vi "DSDLL Cleanup Digitizing Process.vi"(8 "error in":errorcluster, 11 "dsdll in":T1) -> (0 "error out":errorcluster, 3 "dsdll out":T1)   [LabVIEW 2018, in "DSDLL Virtual Digitizer.lvlib"]
doc: "Cleans up everything related to the digitizing process. Must be called after each use of Initiate Digitizing Process to deallocate all related objects and to stop Digitizing Process. It must be called even if digitizing failed or was aborted!\nThe VI ignores input error so it will always execute."
uses:
  DSDLL Virtual Digitizer.lvlib
  DSDLL Session.ctl
  dsdll source distribution/dsdll_instance.ctl
  dsdll source distribution/dsdll_device_record.ctl
  DSDLL Process Config.ctl
  DSDLL Data Packet.ctl
  dsdll source distribution/dsdll.lvlib
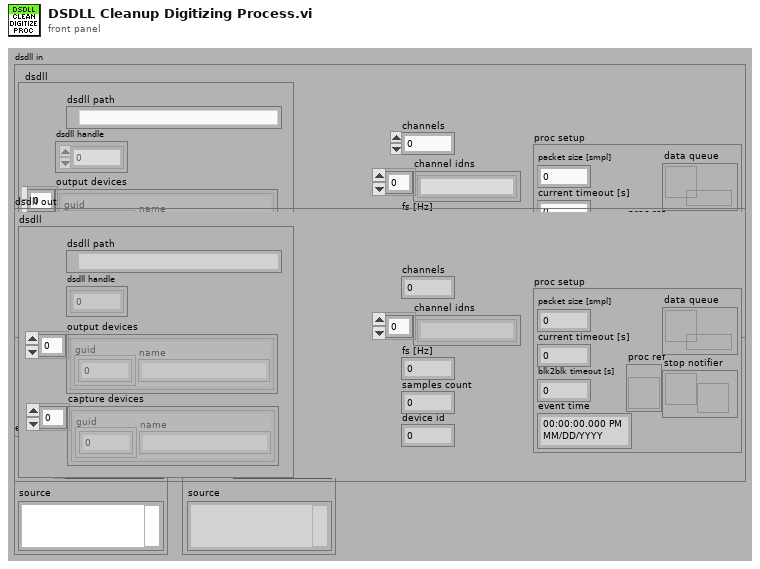
[diagram p1: front panel]
types:
  T1 = typedef "DSDLL Virtual Digitizer.lvlib/DSDLL Session.ctl" = cluster{"dsdll":T2, "channels":i32, "device id":i32, "channel idns":string[], "proc setup":T4, "samples count":i32, "fs [Hz]":dbl}
  T2 = typedef "dsdll.lvlib/dsdll_instance.ctl" = cluster{"dsdll path":path, "dsdll handle":u8[], "output devices":T3[], "capture devices":T3[]}
  T3 = typedef "dsdll.lvlib/dsdll_device_record.ctl" = cluster{"guid":u8[], "name":string}
  T4 = typedef "DSDLL Virtual Digitizer.lvlib/DSDLL Process Config.ctl" = cluster{"packet size [smpl]":i32, "current timeout [s]":dbl, "blk2blk timeout [s]":dbl, "event time":timestamp, "data queue":refnum<queue>, "stop notifier":refnum<notifier>, "proc ref":refnum<vi>}
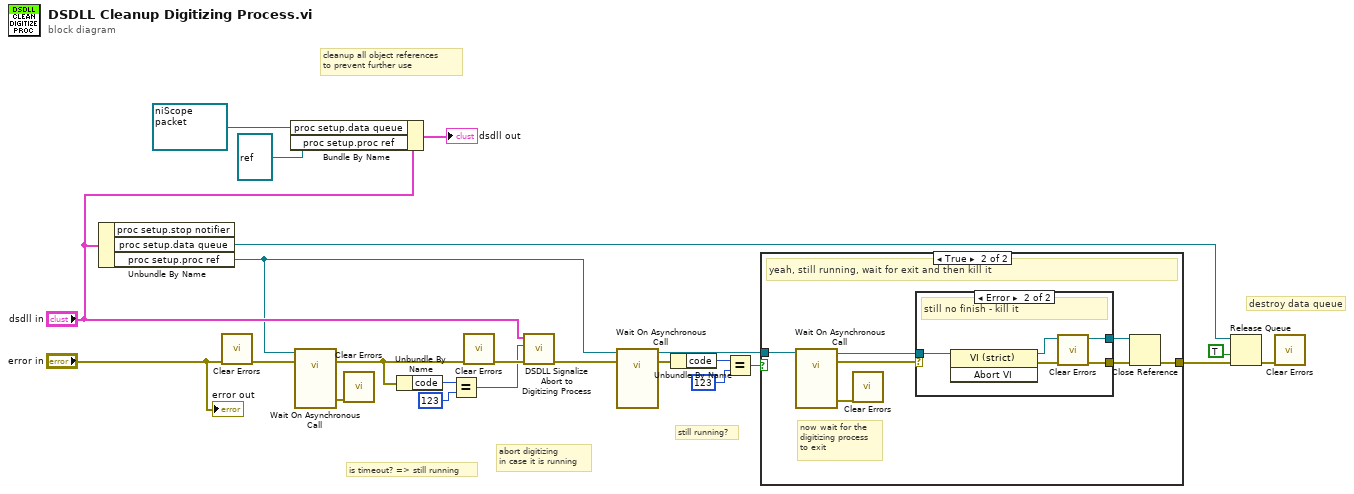
[diagram p0: block diagram]
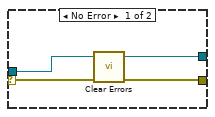
[diagram p3: hidden frame]
diagram:
  # "still running?"
  # "abort digitizing\nin case it is running"
  # "cleanup all object references\nto prevent further use"
  # "destroy data queue"
  # "is timeout? => still running"
  n1 = Unbundle By Name("dsdll in") -> ("proc setup.data queue"=w20:refnum<queue>, "proc setup.proc ref"=w7:refnum<vi>)  [unwired: 1 out]
  n2 = call <vilib>:"Clear Errors.vi"("error in (no error)"="error in") -> ("error out"=w14:errorcluster)  [unwired: 5 in, 1 out]
  n3 = Bundle By Name(cluster="dsdll in", "proc setup.data queue"=refnum<queue> refnum, "proc setup.proc ref"=refnum<vi> refnum) -> (→"dsdll out":T1)
  n4 = call-by-ref "Wait On Asynchronous Call"(reference=w7, error in=w14) -> (error out=w12:errorcluster, 0:"error out"=w13:errorcluster)  [unwired: 10 in, 2 out]
  n5 = call <vilib>:"Clear Errors.vi"("error in (no error)"=w13) -> ()  [unwired: 5 in, 2 out]
  n6 = Unbundle By Name(w12) -> ("code"=w11:i32)
  n7 = Equal?(x=w11, y=123) -> (x = y?=w9:bool)
  n8 = call <vilib>:"Clear Errors.vi"("error in (no error)"=w12) -> ("error out"=w23:errorcluster)  [unwired: 5 in, 1 out]
  n9 = call "DSDLL Signalize Abort to Digitizing Process.vi"("error in"=w23, "send abort signal? (True)"=w9, "dsdll in"="dsdll in") -> ("error out (copy)"=w8:errorcluster)  [unwired: 7 in, 1 out]
  n10 = call-by-ref "Wait On Asynchronous Call"(reference=w7, error in=w8) -> (reference out=w2:refnum<vi>, error out=w6:errorcluster)  [unwired: 10 in, 2 out]
  n11 = Unbundle By Name(w6) -> ("code"=w5:i32)
  n12 = Equal?(x=w5, y=123) -> (x = y?=w3:bool)
  n13 = case shown="True" w3 {
    tunnel: [_ w25] -> w19
    tunnel: w2 -> [_ w27]
    frame False {
    }
    frame True {
      # "now wait for the\ndigitizing process\nto exit"
      # "yeah, still running, wait for exit and then kill it"
      n14 = call-by-ref "Wait On Asynchronous Call"(reference=w27) -> (reference out=w29:refnum<vi>, error out=w30:errorcluster, 0:"error out"=w28:errorcluster)  [unwired: 11 in, 1 out]
      n15 = call <vilib>:"Clear Errors.vi"("error in (no error)"=w28) -> ()  [unwired: 5 in, 2 out]
      n16 = case shown="Error" w30 {
        selector: w30 -> [w32 _]
        tunnel: w29 -> [w31 w37]
        tunnel: [w33 w35] -> w26
        tunnel: [w31 w34] -> w24
        frame No Error {
          n17 = call <vilib>:"Clear Errors.vi"("error in (no error)"=w32) -> ("error out"=w33:errorcluster)  [unwired: 5 in, 1 out]
        }
        frame Error {
          # "still no finish - kill it"
          n18 = invoke class="VI (strict)" method="Abort VI"(reference=w37) -> (reference out=w34:refnum<vi>, error out=w36:errorcluster)  [unwired: 2 in, 1 out]
          n19 = call <vilib>:"Clear Errors.vi"("error in (no error)"=w36) -> ("error out"=w35:errorcluster)  [unwired: 5 in, 1 out]
        }
      }
      n20 = Close Reference(reference=w24, error in (no error)=w26) -> (error out=w25:errorcluster)
    }
  }
  n21 = Release Queue(queue=w20, force destroy? (F)=TRUE, error in (no error)=w19) -> (error out=w22:errorcluster)  [unwired: 2 out]
  n22 = call <vilib>:"Clear Errors.vi"("error in (no error)"=w22) -> ()  [unwired: 5 in, 2 out]
  "error out" <- "error in"
